vi "Aquire XBox Controller Data.vi"(0 "Device ID In":refnum<k1>, 3 "Error In":errorcluster) -> (1 "Device ID Out":refnum<k1>, 4 "Error Out":errorcluster, 5 "Axis Info":T3, 6 "Button Info":T2, 7 "Direction Info":T1)   [LabVIEW 2011]
uses:
  <vilib>/Utility/inputDevices.llb/joystickAcquire.vi
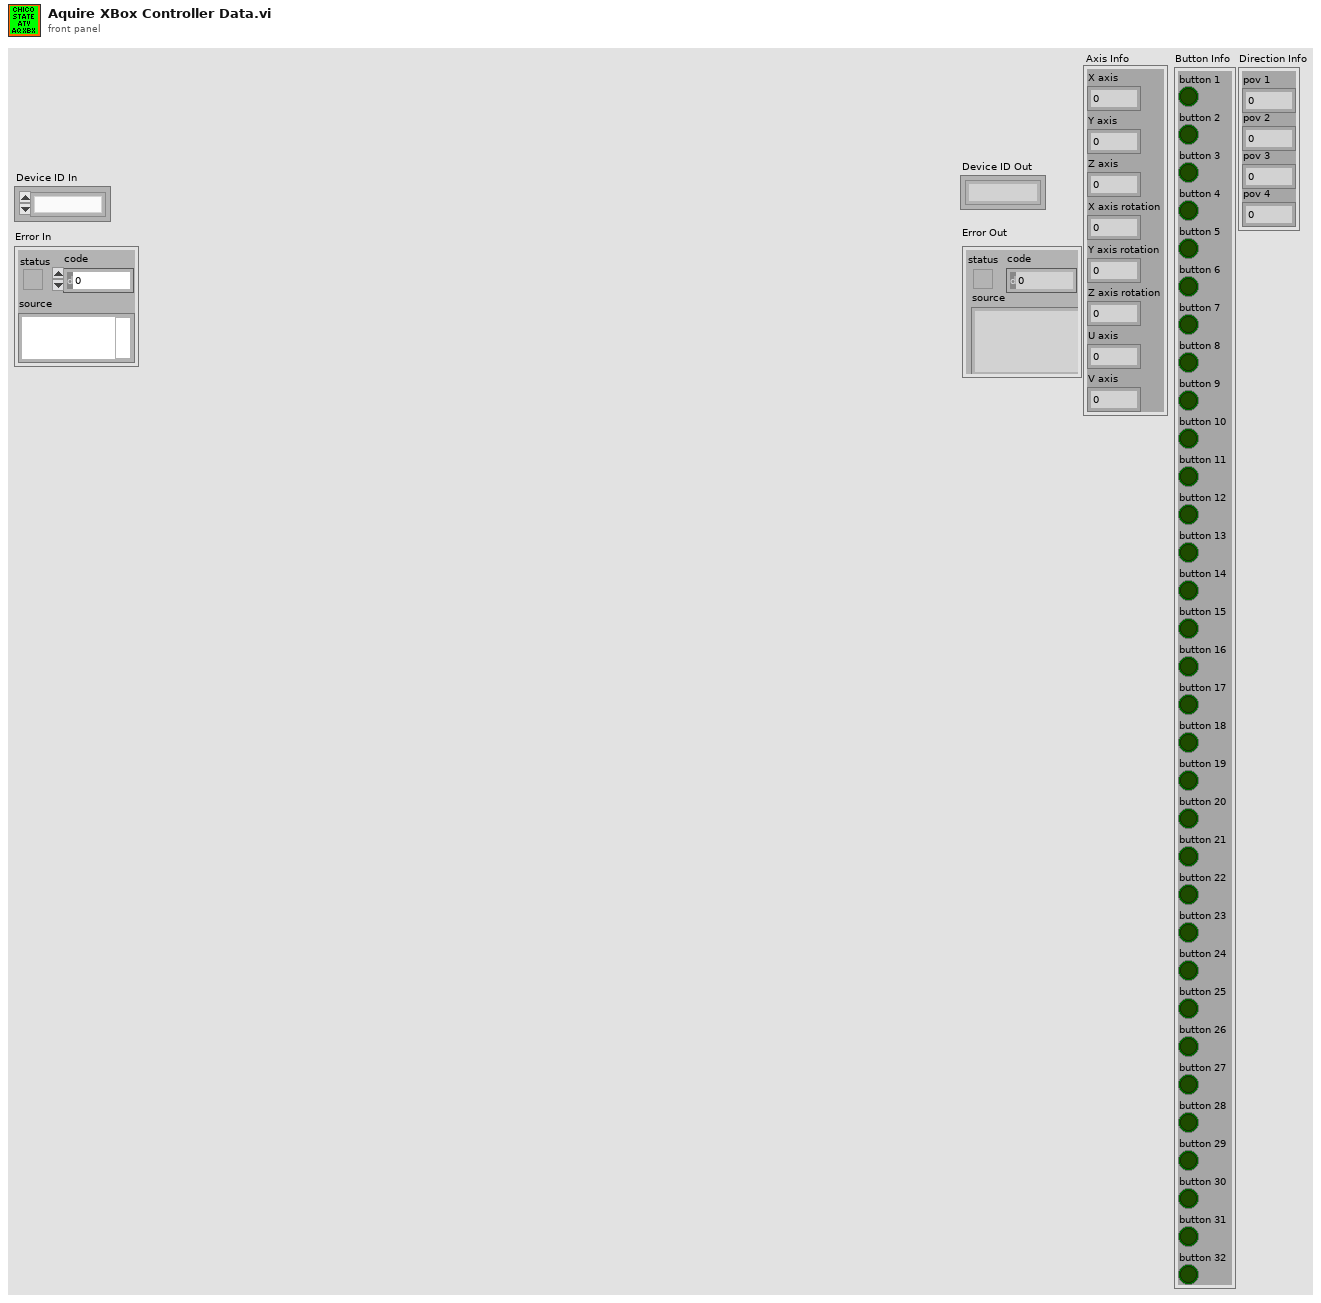
[diagram p1: front panel]
types:
  T1 = cluster{"pov 1":i32, "pov 2":i32, "pov 3":i32, "pov 4":i32}
  T2 = cluster{"button 1":bool, "button 2":bool, "button 3":bool, "button 4":bool, "button 5":bool, "button 6":bool, "button 7":bool, "button 8":bool, "button 9":bool, "button 10":bool, "button 11":bool, "button 12":bool, "button 13":bool, "button 14":bool, "button 15":bool, "button 16":bool, "button 17":bool, "button 18":bool, "button 19":bool, "button 20":bool, "button 21":bool, "button 22":bool, "button 23":bool, "button 24":bool, "button 25":bool, "button 26":bool, "button 27":bool, "button 28":bool, "button 29":bool, "button 30":bool, "button 31":bool, "button 32":bool}
  T3 = cluster{"X axis":i32, "Y axis":i32, "Z axis":i32, "X axis rotation":i32, "Y axis rotation":i32, "Z axis rotation":i32, "U axis":i32, "V axis":i32}
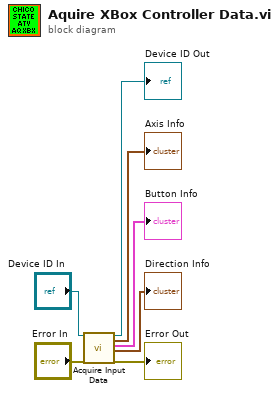
[diagram p0: block diagram]
diagram:
  n1 = call-poly <vilib>:"Acquire Input Data.vi"("device ID"="Device ID In", "error in (no error)"="Error In") -> ("device ID"=→"Device ID Out":refnum<k1>, "axis info"=→"Axis Info":T3, "button info"=→"Button Info":T2, "direction info"=→"Direction Info":T1, "error out"=→"Error Out":errorcluster)  [unwired: 13 in]
